vi "Tag Metadata Sort Tags.vi"(7 "Tags":string[](array[string])=["test", "testing", "Tester", "Apple", "appeal", "annoy", "lead", "Leed", "Lard", "Lean", "learn", "yo", "yoyo", "You", "your", "yours", "cat", "came", "couple", "001", "02", "0101", "123", "45", "65", "87", "86", "83", "99", "91"]) -> (4 "Sorted Tags":string[](array[string]), 8 "First Letters":string[](array[string]), 15 "Letter Indicies":i32[](array[numeric]))   [LabVIEW 2020]
uses:
  <vilib>/Utility/error.llb/whitespace.ctl
  a1cd6b26-20b5-4310-a215-defcd438fa2a.vi
  <vilib>/Array/Sort 2D Array - Pop Stack.vi
  <vilib>/Array/Sort 2D Array - Push Stack.vi
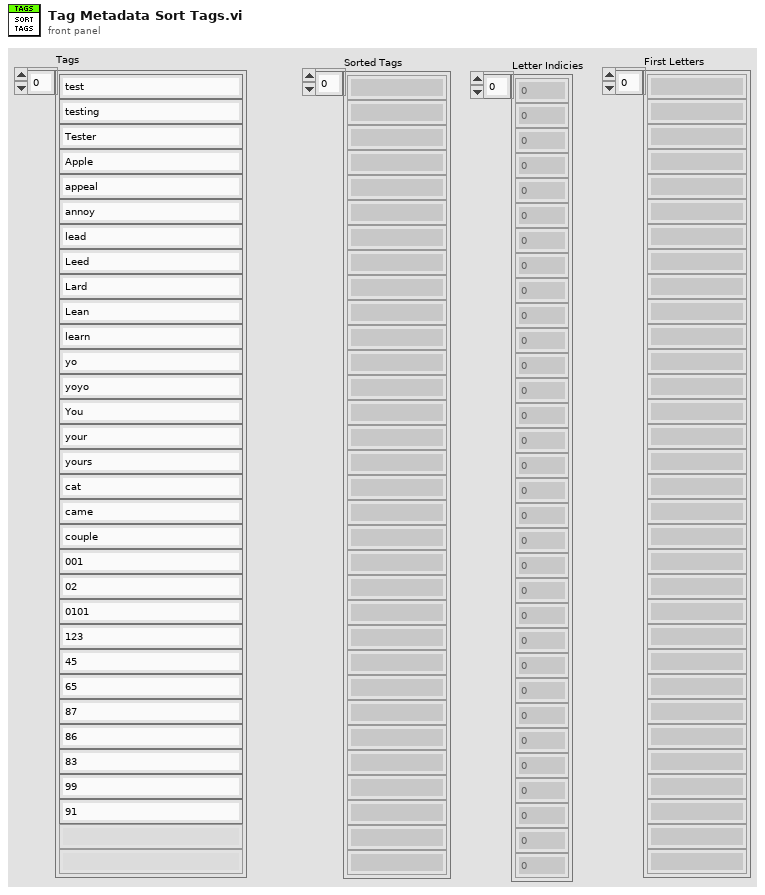
[diagram p1: front panel]
types:
  T1 = typedef "whitespace.ctl" = u16
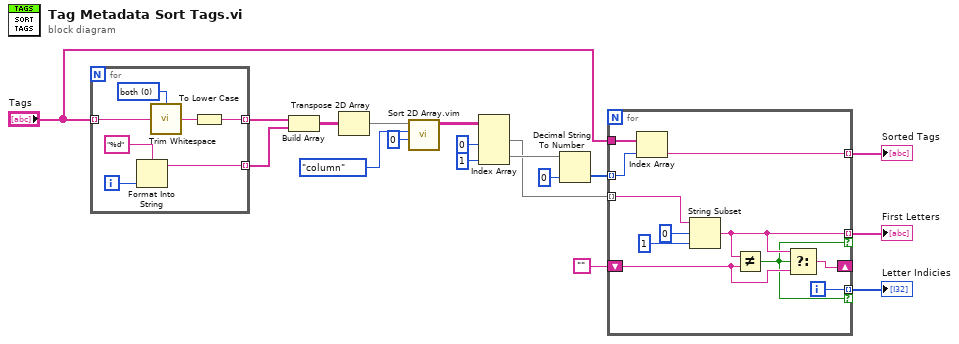
[diagram p0: block diagram]
diagram:
  n1 = for {
    tunnel: "Tags" -> [w25] mode=indexing
    tunnel: [w22] -> w18 mode=indexing
    tunnel: [w19] -> w17 mode=indexing
    i -> [w21]
    w24 = T1 0 items=["both", "start of string", "end of string"] ("location (both)")
    n2 = Format Into String(format string="%d", w21) -> (resulting string=w19:string)  [unwired: 2 in, 1 out]
    n3 = call <vilib>:"Trim Whitespace.vi"("string"=w25, "location (both)"=w24) -> ("trimmed string"=w23:string)
    n4 = To Lower Case(string=w23) -> (all lower case string=w22:string)
  }
  n5 = Build Array(w18, w17) -> (w16:string[][])
  n6 = Transpose 2D Array(2D array=w16) -> (transposed array=w15:string[][])
  n7 = call "Sort 2D Array.vim"("index"=0, "dimension to index (column)"=enum16{"column", "row"}."column", "2D array"=w15) -> ("sorted 2D array"=w12:string[][])  [unwired: 7 in, 1 out]
  n8 = Index Array(array=w12, index (col) #1=0 ("disabled index (col)"), index (col) #2=1 ("index (col)")) -> (element #1=w1:string[], element #2=w9:string[])  [unwired: 2 in]
  n9 = Decimal String To Number(string=w9, default (0L)=0 ("default (0 I32)")) -> (number=w7:i32[])  [unwired: 1 in, 1 out]
  n10 = for {
    tunnel: w7 -> [w29] mode=indexing
    tunnel: "Tags" -> [w36]
    tunnel: [w33] -> w2 mode=indexing
    shift-right: [w31] -> _
    shift-left: "" -> [w32]
    tunnel: [w30] -> w3 mode=indexing if=w26
    tunnel: w1 -> [w28] mode=indexing
    tunnel: [w27] -> w4 mode=indexing if=w26
    i -> [w30]
    n11 = Index Array(array=w36, index=w29) -> (element=w33:string)
    n12 = String Subset(string=w28, offset (0)=0, length (rest)=1 ("length (rest)")) -> (substring=w27:string)
    n13 = Not Equal?(x=w27, y=w32) -> (x != y?=w26:bool)
    n14 = Select(t=w27, s=w26, f=w32) -> (s? t:f=w31:string)
  }
  "Sorted Tags" <- w2
  "Letter Indicies" <- w3
  "First Letters" <- w4
